vi "Engineering mode.vi"() -> ()   [LabVIEW 2017]
uses:
  Ctrls/TesterInfo.ctl
  Ctrls/control_hard.ctl
  Ctrls/HD Config.ctl
  Ctrls/AllControls.ctl
  <vilib>/Utility/miscctls.llb/LVRowAndColumnTypeDef.ctl
  Ctrls/Position Config.ctl
  Thorlabs.MotionControl.IntegratedStepperMotorsCLI.dll
  ComVIS/Files/Ini/WriteIniFiles_ByVarient.vi
  <vilib>/Utility/file.llb/Write Delimited Spreadsheet (string).vi
  HardWare/ADLINK/IO/Adlink IO/Adlink IO.lvlib
  Thorlabs.MotionControl.Controls.dll
panel:
  in  "Production Mode":bool
  out "Boolean":bool=TRUE
  in  "SerialNumber":string
  in  "Data":string
  out "Size":i32
  in  "AllControls":T1
  out "Save_status":string
  in  "Selecttion":T2(tab)
  in  "HD Config 2":T3
  in  "HD Config Save":bool
  in  "HD Config":T3
  in  "SW Config Save":bool
  in  "TesterInfo":T4={"Station Name"="", "Station Code"="", "ES NO."="", "Tester ID"="", "PassMark Revision"="", "Rig ID"="", "682_Tool_Repeat"="12", "Project Name"="", "FFTesterPath"=path "", "Enable_User"=FALSE, "Mode"=enum."682", "Fail_resume_mode"=FALSE}
  in  "Table":T5(tab)
  in  "Table_Data":string[][](table)
  in  "Title_Data":string[][](table)
  in  "Config":string[][](table)
  in  "SKU_Table":string[][](table)
  in  "Debug":T6
  in  "IO":i32(listbox)
  in  "LongTravelStageControl":refnum<k24>(container)
  in  "MoveAbsolute2":bool
  in  "MoveAbsolute1":bool
  in  "White":dbl=60.0 max=150.0
  in  "Home":bool
  in  "Black":dbl=30.0 max=150.0
  in  "Position Config Save":bool
  out "LedValue":string
  in  "Led_Read":bool
  out "Led Data":string
  out "standard output":string
  in  "SendCMD":bool
  in  "NFC_Connect":bool
  out "NFC_Connected":string
  in  "682_Tool_CMD":T7(ring)
  out "temperature":dbl
  out "humidity":dbl
  in  "ReadTemp&Hum":bool
  out "Res Data":string
  # "Unit: mm"
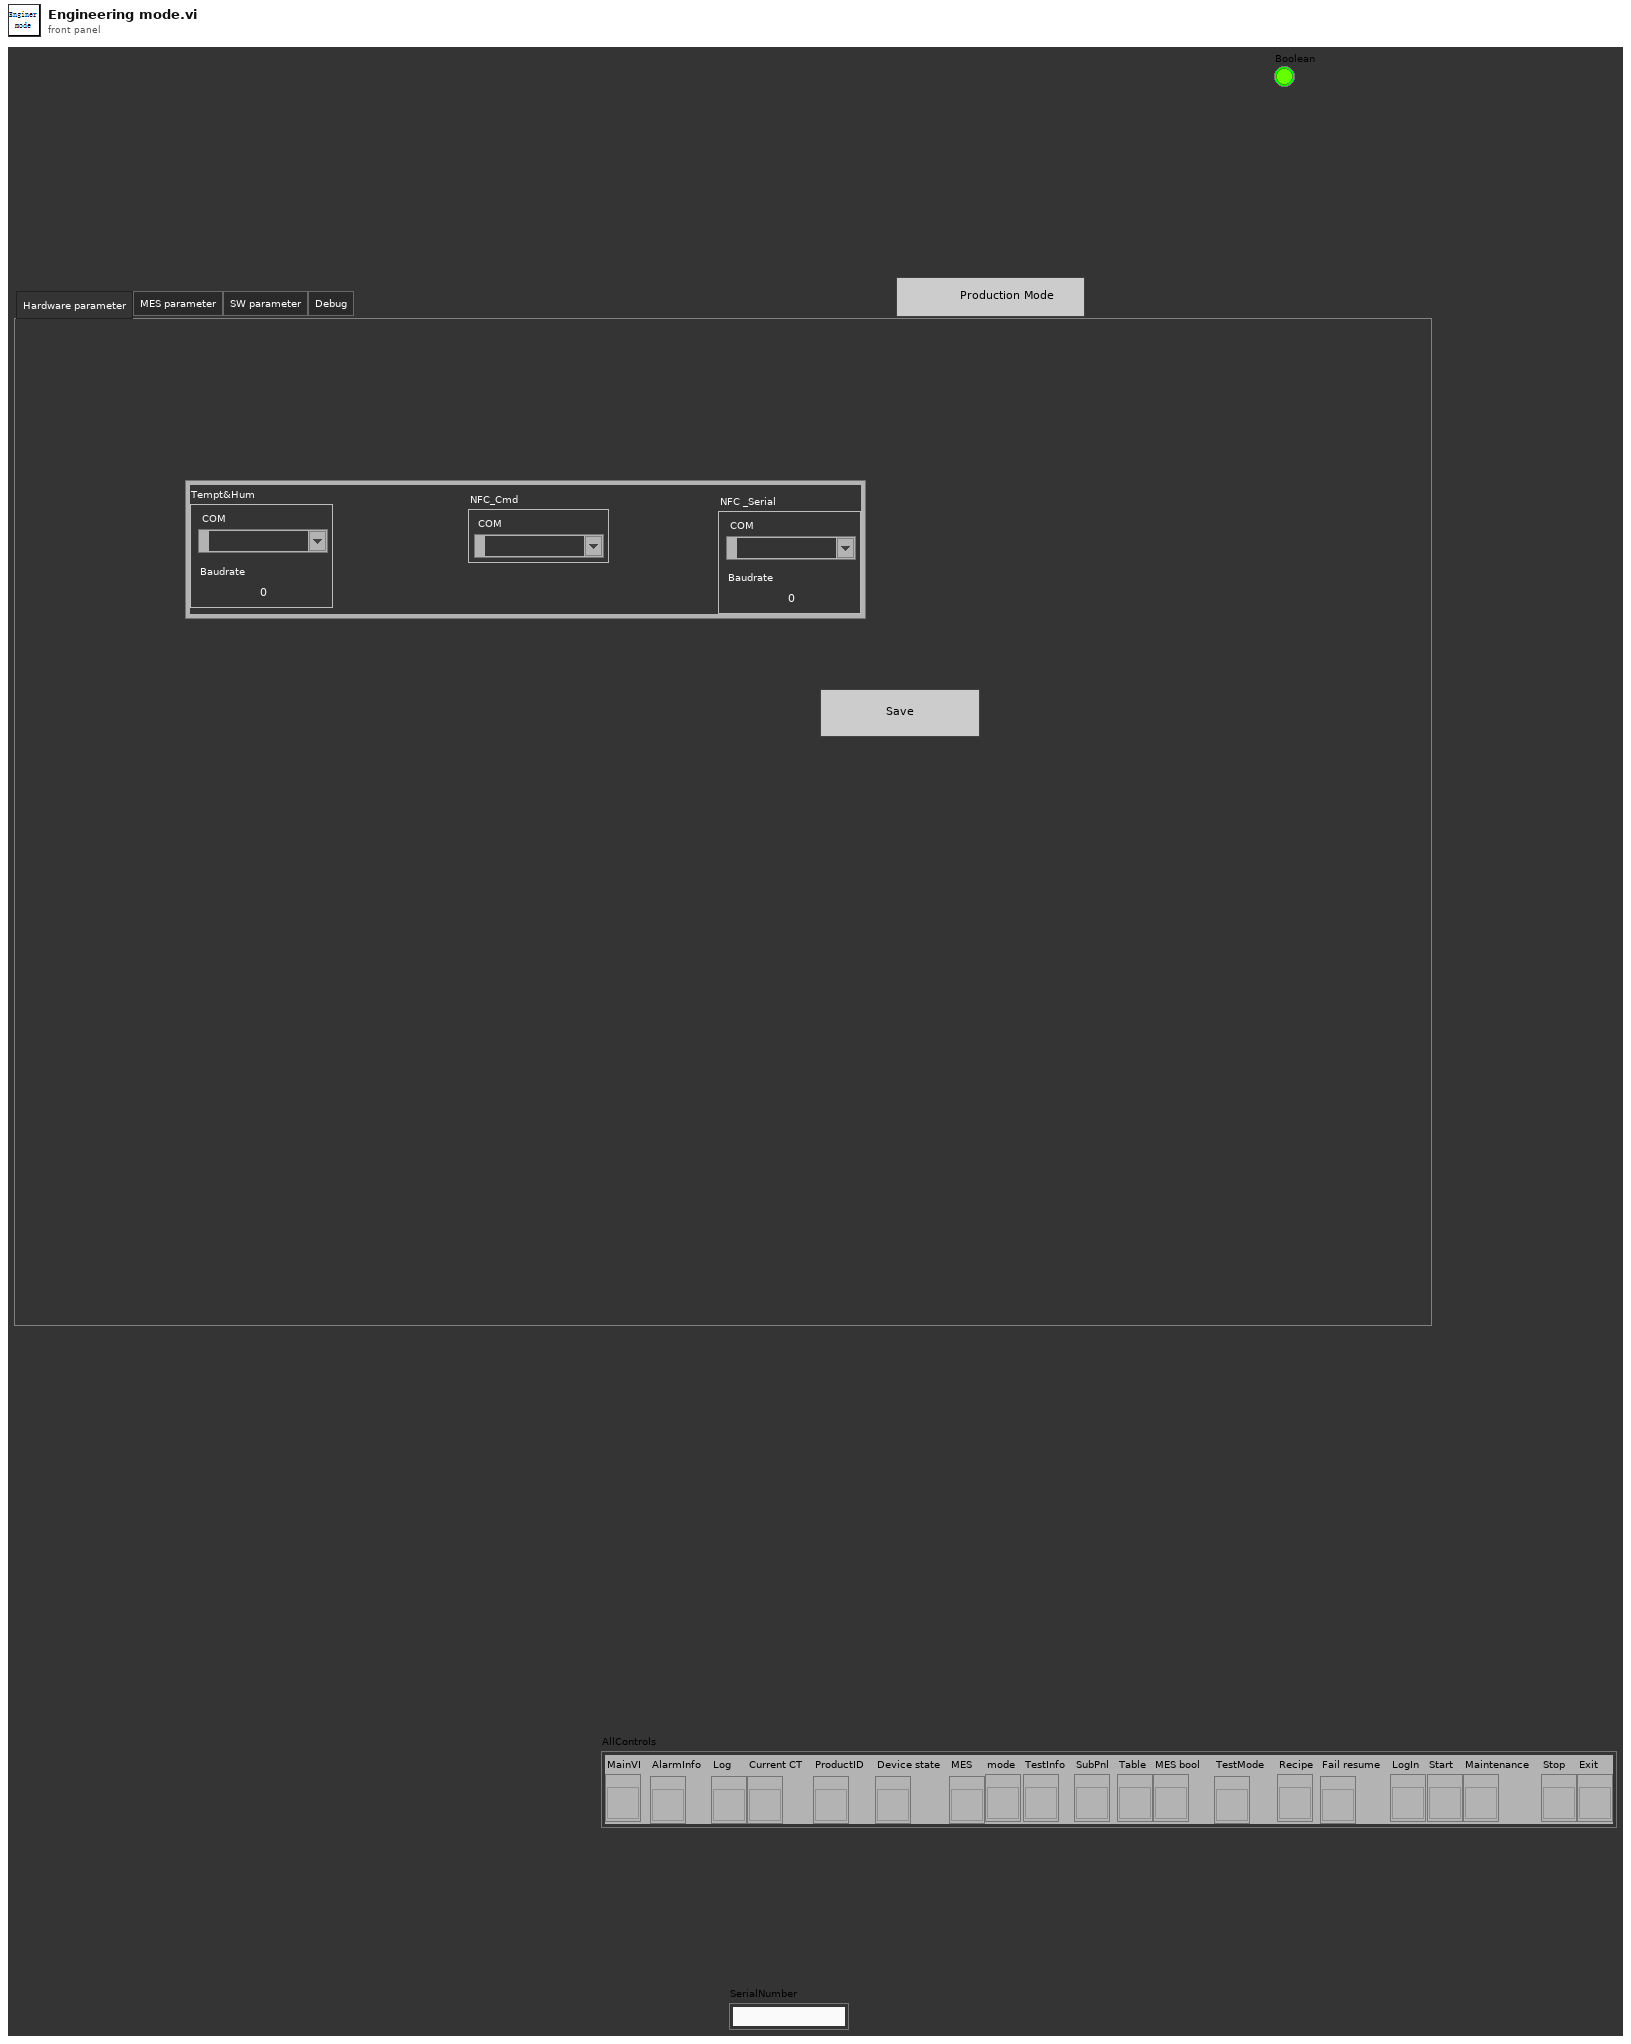
[diagram p1: front panel]
types:
  T1 = typedef "AllControls.ctl" = cluster{"MainVI":refnum<vi>, "AlarmInfo":refnum<vi>, "Log":refnum<vi>, "Current CT":refnum<vi>, "ProductID":refnum<vi>, "Device state":refnum<vi>, "MES":refnum<vi>, "mode":refnum<vi>, "TestInfo":refnum<vi>, "SubPnl":refnum<vi>, "Table":refnum<vi>, "MES bool":refnum<vi>, "TestMode":refnum<vi>, "Recipe":refnum<vi>, "Fail resume":refnum<vi>, "LogIn":refnum<vi>, "Start":refnum<vi>, "Maintenance":refnum<vi>, "Stop":refnum<vi>, "Exit":refnum<vi>}
  T2 = enum32{"Hardware parameter", "MES parameter", "SW parameter", "Debug"}
  T3 = typedef "HD Config.ctl" = cluster{" PC":cluster{"PC Address":u8[], "PC Port":i32}, "FCO":cluster{"COM":refnum<visa-resource-name>, "Baudrate":u32}, "DC Power ":cluster{"COM":refnum<visa-resource-name>, "Baudrate":u32}, "PW3336":cluster{"COM":refnum<visa-resource-name>, "Baudrate":u32}, "Lefoo":cluster{"COM":refnum<visa-resource-name>, "Baudrate":u32}, "Tempt&Hum":cluster{"COM":refnum<visa-resource-name>, "Baudrate":u32}, "DIPC":cluster{"COM":refnum<visa-resource-name>}, "Daemon":cluster{"IP Address":string, "Port":u16, "Retry":u16}, "NFC_Cmd":cluster{"COM":refnum<visa-resource-name>, "Baudrate":u32}, "Fail_resume_mode":bool, "GRR":bool, "NFC _Serial":cluster{"COM":refnum<visa-resource-name>, "Baudrate":u32}}
  T4 = typedef "TesterInfo.ctl" = cluster{"Station Name":string, "Station Code":string, "ES NO.":string, "Tester ID":string, "PassMark Revision":string, "Rig ID":string, "682_Tool_Repeat":string, "Project Name":string, "FFTesterPath":path, "Enable_User":bool, "Mode":enum16{"682"}, "Fail_resume_mode":bool}
  T5 = enum32{"Process_parameter_Setting", "Passmark_Setting", "Setting_Config", "SKU_Table"}
  T6 = typedef "control_hard.ctl" = enum32{"IO Control", "Motor_Plate control", "Led Read", "NFC ", "PW3336_Power Meter", "Lefoo_Atm Pressure", "Temp&Hum", "Set EOL_URAT"}
  T7 = enum16{"Start Test Mode", "Getting Software Version", "Start camera test mode", "Get one image", "Stop camera test mode", "Stop Test Mode", "Get image uniformity andFlash LED brightness", "Get image reflection", "Enable flash LED", "Disable flash LED", "Tune Flash LED brightness", "Start Camera calibration", "Software Reset", "Verify OBC Setting"}
  T8 = cluster{"COM":refnum<visa-resource-name>, "Baudrate":u32}
  T9 = cluster{"DI dev":i32[], "DI line":i32[], "Port":i32[], "DO dev":i32[], "DO line":i32[], "IO Data":string[][], "IO f":i16[]}
  T10 = typedef "amc_Message Queue.ctl" = refnum<queue>
  T11 = typedef "LVRowAndColumnTypeDef.ctl" = cluster{"Row":i32, "Column":i32}
  T12 = typedef "LVPoint32TypeDef.ctl" = cluster{"Horizontal":i32, "Vertical":i32}
  T13 = enum8{"Enabled", "Disabled", "Disabled and Grayed Out"}
  T14 = typedef "Position Config.ctl" = cluster{"Black":dbl, "White":dbl, "Black1":dbl, "White1":dbl}
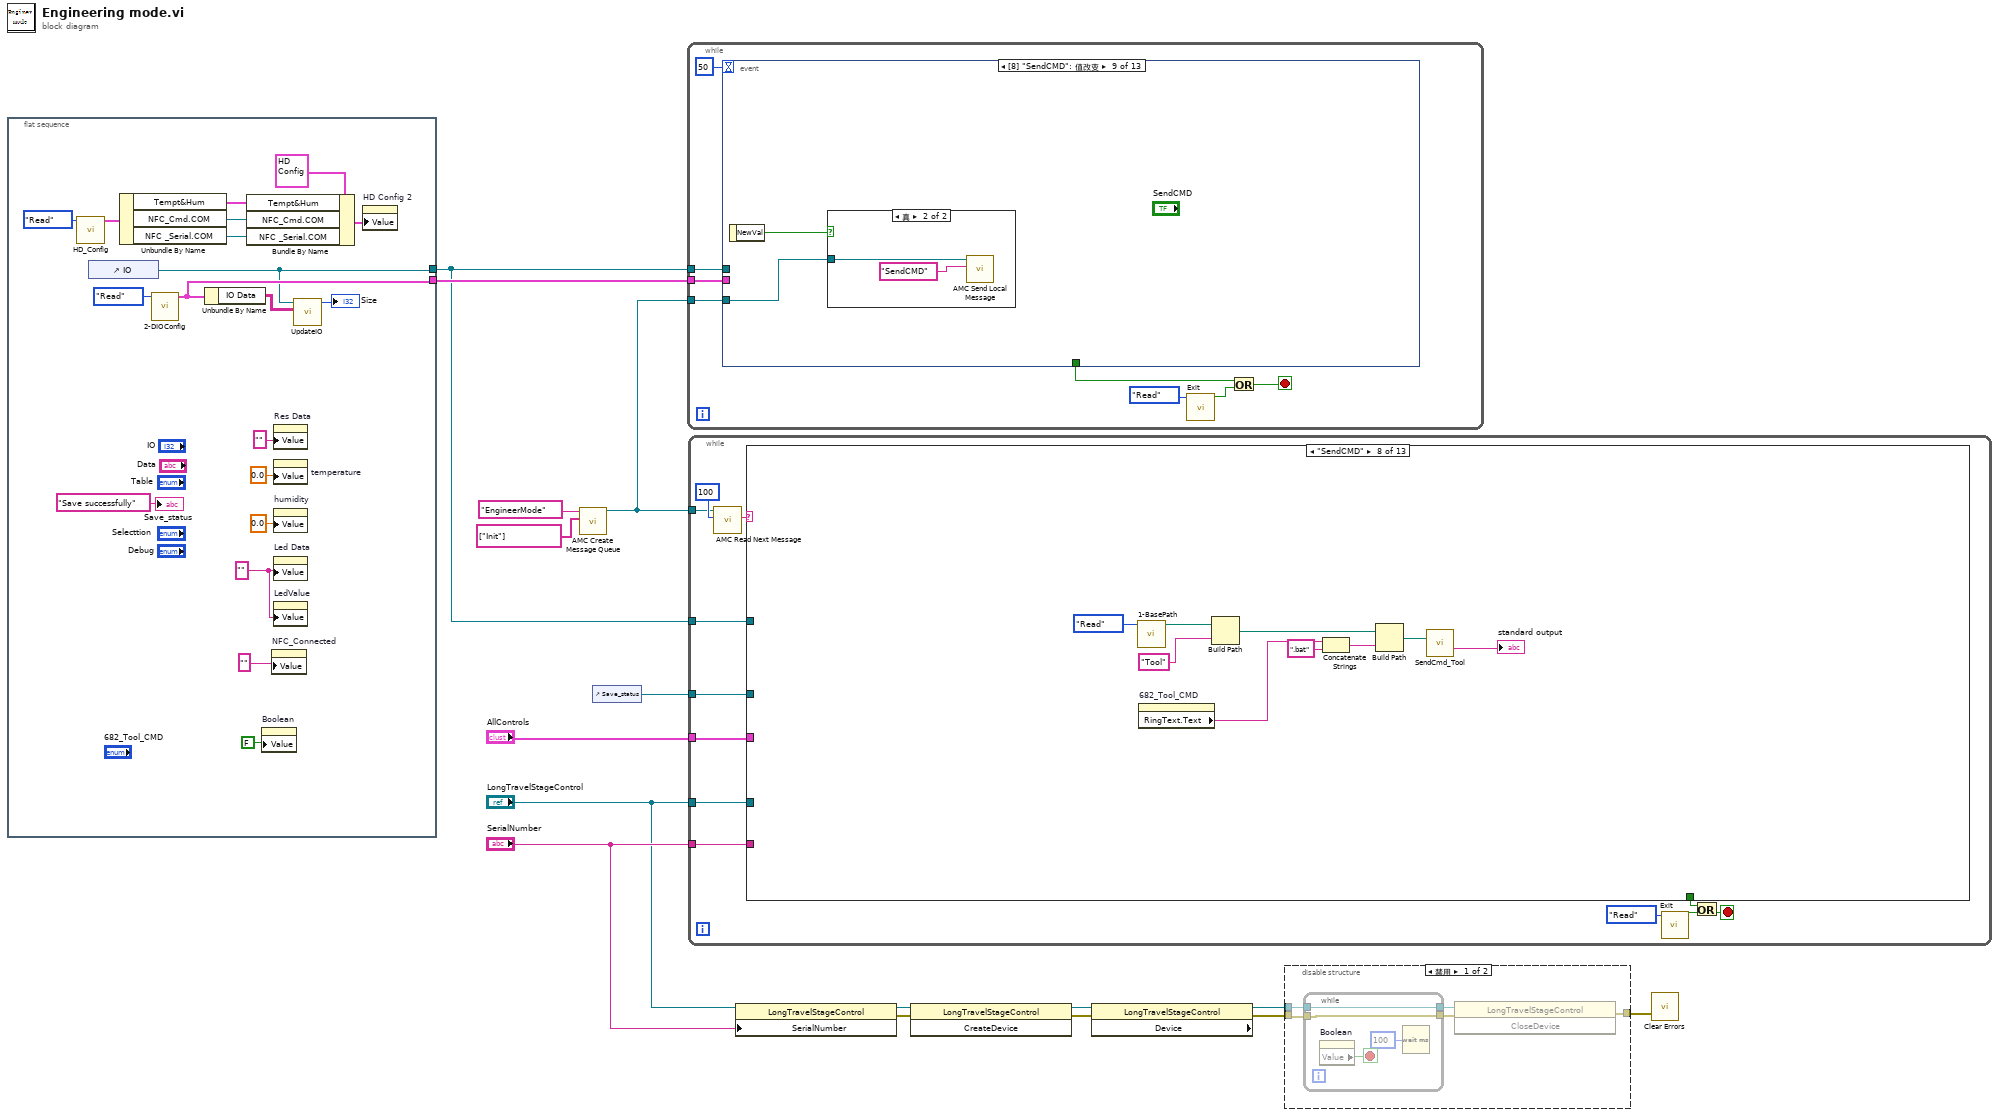
[diagram p0: block diagram]
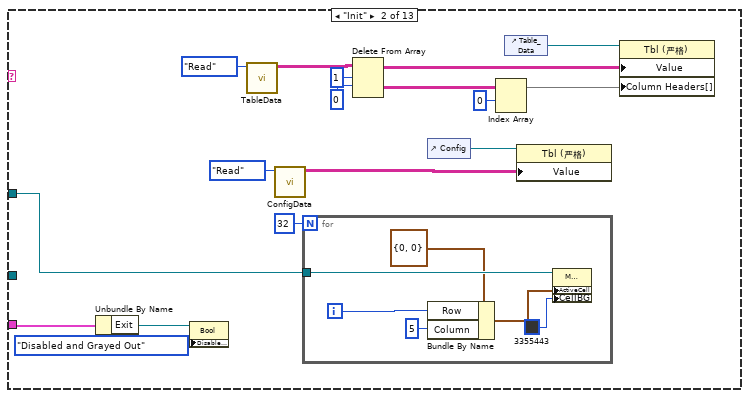
[diagram p4: hidden frame]
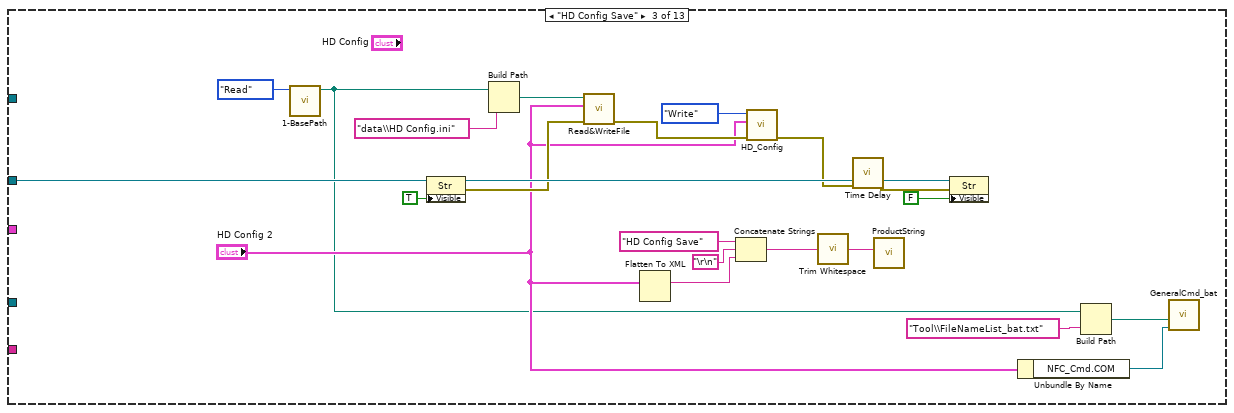
[diagram p5: hidden frame]
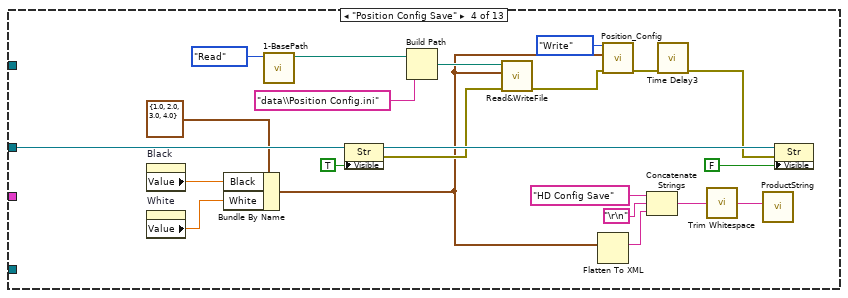
[diagram p6: hidden frame]
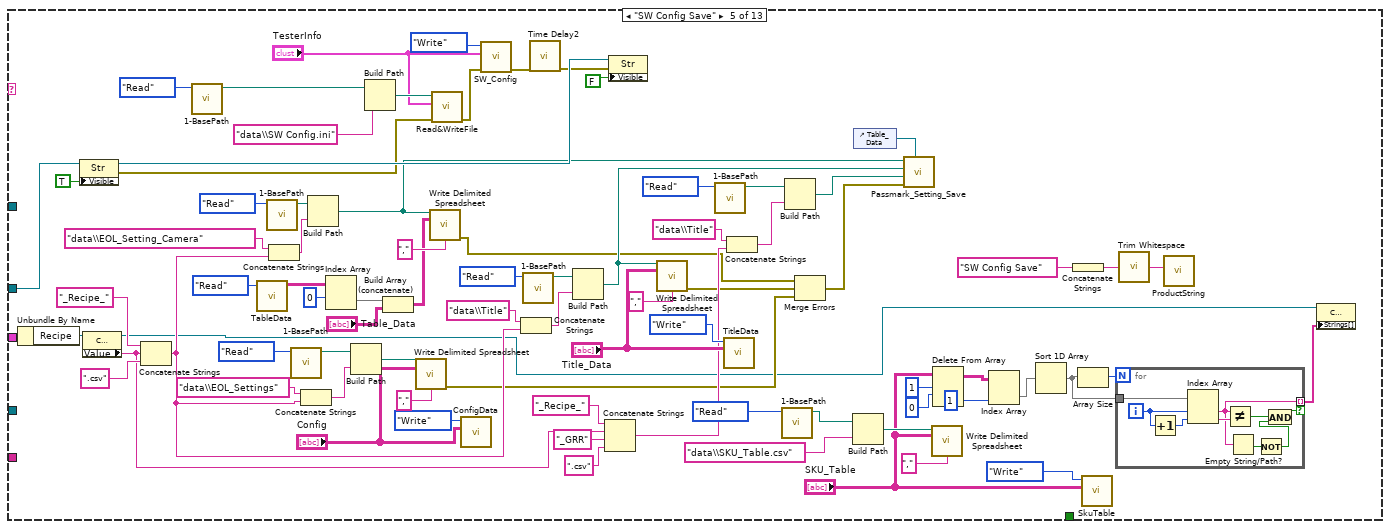
[diagram p7: hidden frame]
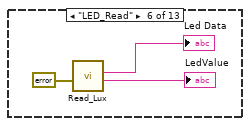
[diagram p8: hidden frame]
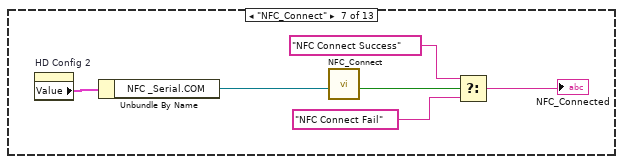
[diagram p9: hidden frame]
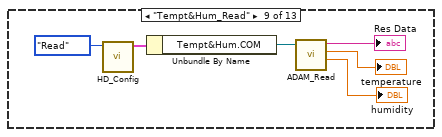
[diagram p10: hidden frame]
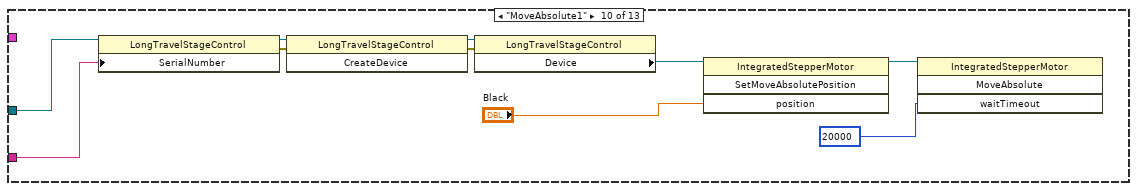
[diagram p11: hidden frame]
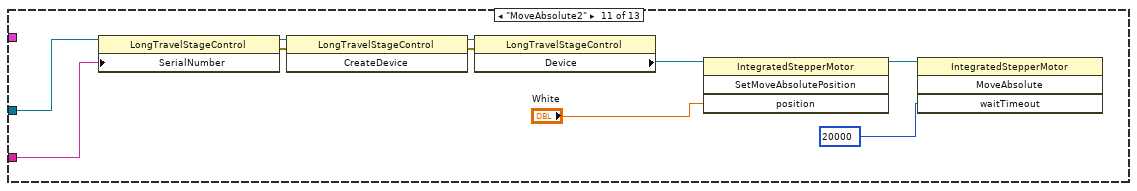
[diagram p12: hidden frame]
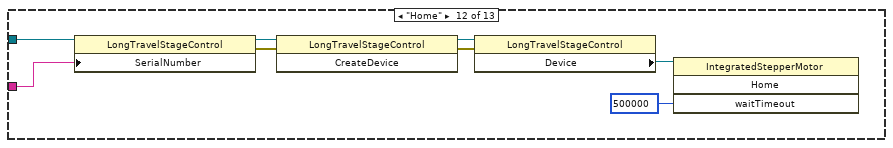
[diagram p13: hidden frame]
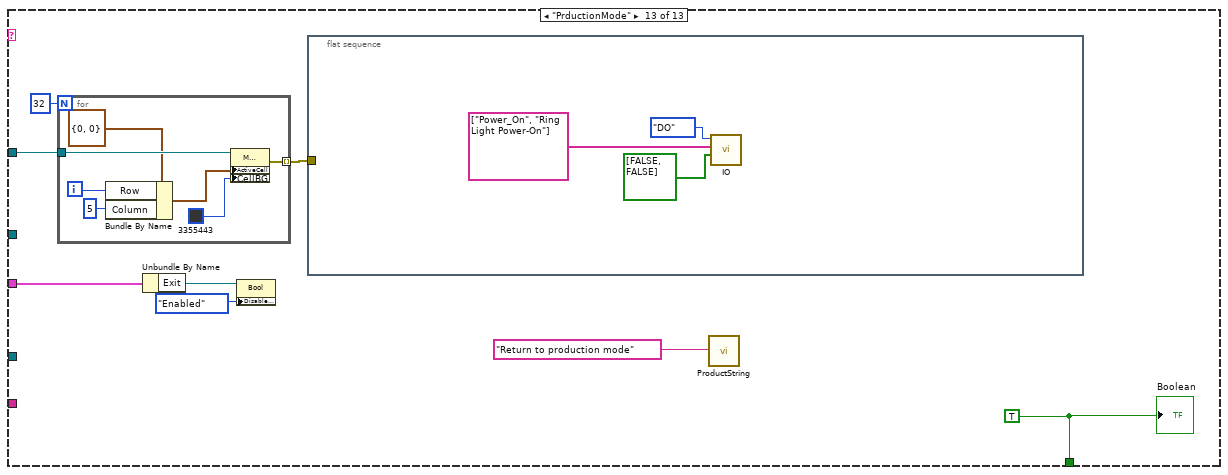
[diagram p14: hidden frame]
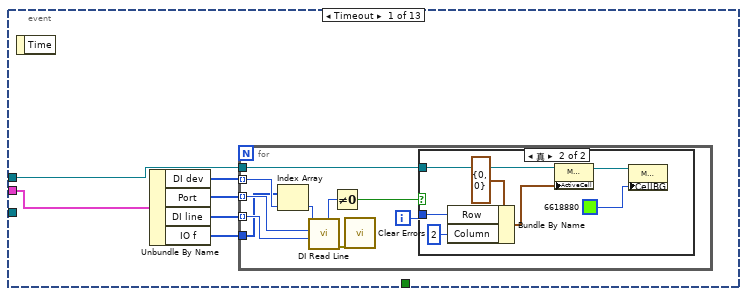
[diagram p15: hidden frame]
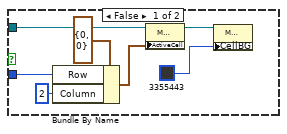
[diagram p16: hidden frame]
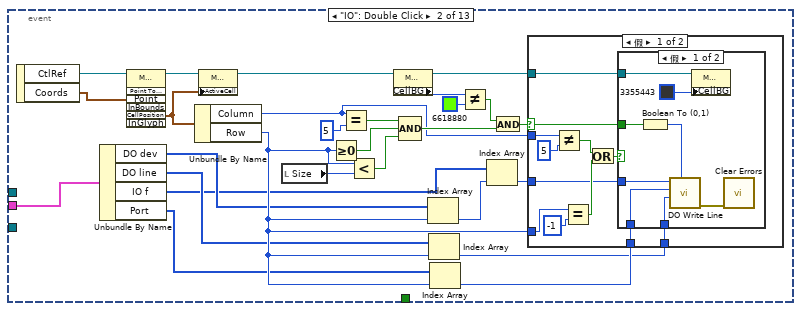
[diagram p17: hidden frame]
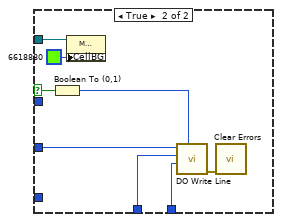
[diagram p19: hidden frame]
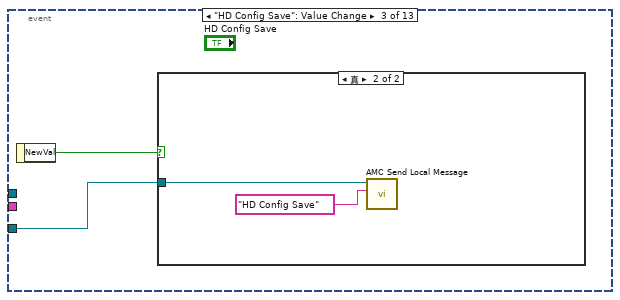
[diagram p20: hidden frame]
diagram:
  n1 = flat-sequence {
    tunnel: [w33] -> w11
    tunnel: [w31] -> w10
    frame #0 {
      w21 = "" ("Led Data")
      n2 = call "HD_Config.vi"("Step"=enum16{"Initial", "Write", "Read"}."Read") -> ("HD Config out"=w29:T3)  [unwired: 9 in, 1 out]
      n3 = control-ref of="IO"() -> (w31:refnum<vi>)
      n4 = Unbundle By Name(w29) -> ("Tempt&Hum"=w26:T8, "NFC_Cmd.COM"=w20:refnum<visa-resource-name>, "NFC _Serial.COM"=w18:refnum<visa-resource-name>)
      n5 = call "2-DIOConfig.vi"("Step"=enum16{"Initial", "Write", "Read"}."Read") -> ("DIO pra out"=w33:T9)  [unwired: 9 in, 1 out]
      n6 = Unbundle By Name(w33) -> ("IO Data"=w32:string[][])
      n7 = Bundle By Name(cluster=T3 {" PC"={"PC Address"=[], "PC Port"=0}, "FCO"={"COM"="", "Baudrate"=0}, "DC Power "={"COM"="", "Baudrate"=0}, "PW3336"={"COM"="", "Baudrate"=0}, "Lefoo"={"COM"="", "Baudrate"=0}, "Tempt&Hum"={"COM"="", "Baudrate"=0}, "DIPC"={"COM"=""}, "Daemon"={"IP Address"="", "Port"=0, "Retry"=0}, "NFC_Cmd"={"COM"="", "Baudrate"=0}, "Fail_resume_mode"=FALSE, "GRR"=FALSE, "NFC _Serial"={"COM"="", "Baudrate"=0}} ("HD Config 2"), "Tempt&Hum"=w26, "NFC_Cmd.COM"=w20, "NFC _Serial.COM"=w18) -> (w25:T3)
      n8 = property on="Boolean" class="Bool (严格)"("Value"=FALSE ("Boolean")) -> ()  [unwired: 2 in, 2 out]
      n9 = property on="NFC_Connected" class="Str"("Value"="" ("concatenated string")) -> ()  [unwired: 2 in, 2 out]
      n10 = property on="Res Data" class="Str"("Value"="" ("Res Data")) -> ()  [unwired: 2 in, 2 out]
      n11 = property on="temperature" class="DigNum (严格)"("Value"=0.0 ("temperature")) -> ()  [unwired: 2 in, 2 out]
      n12 = property on="humidity" class="DigNum (严格)"("Value"=0.0 ("humidity")) -> ()  [unwired: 2 in, 2 out]
      n13 = property on="Led Data" class="Str"("Value"=w21) -> ()  [unwired: 2 in, 2 out]
      n14 = property on="LedValue" class="Str"("Value"=w21) -> ()  [unwired: 2 in, 2 out]
      n15 = call "UpdateIO.vi"("IO Data"=w32, "MulticolumnListbox输入"=w31) -> ("大小"=→"Size":i32)  [unwired: 9 in]
      n16 = property on="HD Config 2" class="Clust (严格)"("Value"=w25) -> ()  [unwired: 2 in, 2 out]
      "Save_status" <- "Save successfully" ("Save_status")
    }
  }
  n17 = call "AMC Create Message Queue.vi"("Initial Message Names"=string[] ["Init"], "Message Queue Name"="EngineerMode" ("Message queue name (unnamed)")) -> ("Message Queue out"=w15:T10)  [unwired: 3 in, 6 out]
  n18 = control-ref of="Save_status"() -> (w14:refnum<vi>)
  n19 = while {
    tunnel: w15 -> [w40]
    tunnel: w10 -> [w38]
    tunnel: w11 -> [w37]
    stop <- w36 stop-if-true
    n20 = event shown="[8] \"SendCMD\": 值改变" {
      selector: _ -> [_ _ _ _ _ _ _ _ _ _ _ _ _]
      dyn-events: _ -> [_ _ _ _ _ _ _ _ _ _ _ _ _]
      timeout: 50 -> [_ _ _ _ _ _ _ _ _ _ _ _ _]
      tunnel: w40 -> [_ _ w130 w133 w138 w143 w150 w154 w158 w161 w165 w169 w174]
      tunnel: [_ _ _ _ _ _ _ _ _ _ _ _ w173] -> w39
      tunnel: w38 -> [w44 _ _ _ _ _ _ _ _ _ _ _ _]
      tunnel: w37 -> [w45 w76 _ _ _ _ _ _ _ _ _ _ _]
      event Timeout {
        n21 = event-data() -> ()  [unwired: 1 in, 1 out]
        n22 = Unbundle By Name(w45) -> ("DI dev"=w46:i32[], "Port"=w47:i32[], "DI line"=w48:i32[], "IO f"=w49:i16[])
        n23 = for {
          tunnel: w44 -> [w55]
          tunnel: w46 -> [w52] mode=indexing
          tunnel: w48 -> [w56] mode=indexing
          tunnel: w47 -> [w53] mode=indexing
          tunnel: w49 -> [w50]
          i -> [w54]
          n24 = Index Array(array=w50, index=w52) -> (element=w51:i16)
          n25 = call "DI Read Line.vi"("Line"=w56, "Port"=w53, "CardNumber"=w51) -> ("error out"=w59:errorcluster, "State out"=w58:u16)  [unwired: 6 in, 1 out]
          n26 = Not Equal To 0?(x=w58) -> (x != 0?=w57:bool)
          n27 = call <vilib>:"Clear Errors.vi"("error in (no error)"=w59) -> ()  [unwired: 5 in, 2 out]
          n28 = case shown="真" w57 {
            tunnel: w54 -> [w61 w70]
            tunnel: w55 -> [w60 w67]
            frame False {
              n29 = Bundle By Name(cluster=T11 {"Row"=0, "Column"=0} ("活动单元格:活动单元格"), "Row"=w61, "Column"=2) -> (w64:T11)
              n30 = property class="MCListbox (严格)"(reference=w60, "ActiveCell"=w64) -> (reference out=w66:refnum<vi>)  [unwired: 1 in, 1 out]
              n31 = property class="MCListbox (严格)"(reference=w66, "CellBG"=u32 3355443) -> ()  [unwired: 1 in, 2 out]
            }
            frame True {
              n32 = Bundle By Name(cluster=T11 {"Row"=0, "Column"=0} ("活动单元格:活动单元格"), "Row"=w70, "Column"=2) -> (w71:T11)
              n33 = property class="MCListbox (严格)"(reference=w67, "ActiveCell"=w71) -> (reference out=w73:refnum<vi>)  [unwired: 1 in, 1 out]
              n34 = property class="MCListbox (严格)"(reference=w73, "CellBG"=u32 6618880) -> ()  [unwired: 1 in, 2 out]
            }
          }
        }
      }
      event "IO": Double Click {
        n35 = event-data() -> ("CtlRef"=w75:refnum<vi>, "Coords"=w74:T12)  [unwired: 1 in]
        n36 = Unbundle By Name(w76) -> ("DO dev"=w81:i32[], "DO line"=w80:i32[], "IO f"=w79:i16[], "Port"=w98:i32[])
        n37 = invoke class="MCListbox (严格)" method="Point To Row Column"(reference=w75, "Point"=w74) -> (reference out=w94:refnum<vi>, "CellPosition"=w85:T11)  [unwired: 5 in, 5 out]
        n38 = Unbundle By Name(w85) -> ("Column"=w82:i32, "Row"=w99:i32)
        n39 = property class="MCListbox (严格)"(reference=w94, "ActiveCell"=w85) -> (reference out=w93:refnum<vi>)  [unwired: 1 in, 1 out]
        n40 = local read "Size"() -> (w84:i32)
        n41 = Greater Or Equal To 0?(x=w99) -> (x >= 0?=w90:bool)
        n42 = Equal?(x=w82, y=5) -> (x = y?=w91:bool)
        n43 = Less?(x=w99, y=w84) -> (x < y?=w83:bool)
        n44 = property class="MCListbox (严格)"(reference=w93) -> (reference out=w86:refnum<vi>, "CellBG"=w88:u32)  [unwired: 1 in, 1 out]
        n45 = Compound Arithmetic op=AND(w91, w90, w83) -> (w92:bool)
        n46 = Index Array(array=w81, index=w99) -> (element=w95:i32)
        n47 = Index Array(array=w80, index=w99) -> (element=w97:i32)
        n48 = Index Array(array=w98, index=w99) -> (element=w100:i32)
        n49 = Not Equal?(x=w88, y=u32 6618880) -> (x != y?=w89:bool)
        n50 = Index Array(array=w79, index=w95) -> (element=w96:i16)
        n51 = And(x=w89, y=w92) -> (x .and. y?=w87:bool)
        n52 = case shown="假" w87 {
          selector: w87 -> [w109 w124]
          tunnel: w86 -> [w112 w128]
          tunnel: w82 -> [w108 _]
          tunnel: w96 -> [w103 w126]
          tunnel: w97 -> [w102 w125]
          tunnel: w99 -> [w104 _]
          tunnel: w100 -> [w101 w121]
          frame False {
            n53 = Not Equal?(x=w108, y=5) -> (x != y?=w105:bool)
            n54 = Equal?(x=w104, y=-1) -> (x = y?=w110:bool)
            n55 = Or(x=w105, y=w110) -> (x .or. y?=w106:bool)
            n56 = case shown="假" w106 {
              tunnel: w112 -> [w119 _]
              tunnel: w109 -> [w114 _]
              tunnel: w103 -> [w115 _]
              tunnel: w102 -> [w116 _]
              tunnel: w101 -> [w113 _]
              frame False {
                n57 = Boolean To (0,1)(Boolean=w114) -> (0, 1=w118:i16)
                n58 = call "DO Write Line.vi"("Value"=w118, "Line"=w116, "Port"=w113, "CardNumber"=w115) -> ("error out"=w117:errorcluster)  [unwired: 6 in, 1 out]
                n59 = property class="MCListbox (严格)"(reference=w119, "CellBG"=u32 3355443) -> ()  [unwired: 1 in, 2 out]
                n60 = call <vilib>:"Clear Errors.vi"("error in (no error)"=w117) -> ()  [unwired: 5 in, 2 out]
              }
              frame True {
              }
            }
          }
          frame True {
            n61 = Boolean To (0,1)(Boolean=w124) -> (0, 1=w123:i16)
            n62 = property class="MCListbox (严格)"(reference=w128, "CellBG"=u32 6618880) -> ()  [unwired: 1 in, 2 out]
            n63 = call "DO Write Line.vi"("Value"=w123, "Line"=w125, "Port"=w121, "CardNumber"=w126) -> ("error out"=w122:errorcluster)  [unwired: 6 in, 1 out]
            n64 = call <vilib>:"Clear Errors.vi"("error in (no error)"=w122) -> ()  [unwired: 5 in, 2 out]
          }
        }
      }
      event "HD Config Save": Value Change {
        n65 = event-data() -> ("NewVal"=w129:bool)  [unwired: 1 in]
        n66 = case shown="真" w129 {
          tunnel: w130 -> [_ w132]
          frame False {
          }
          frame True {
            n67 = call "AMC Send Local Message.vi"("Message Name"="HD Config Save", "Message Queue in"=w132) -> ()  [unwired: 8 in, 2 out]
          }
        }
      }
      event "SW Config Save": Value Change {
        n68 = event-data() -> ("NewVal"=w134:bool)  [unwired: 1 in]
        n69 = case shown="真" w134 {
          tunnel: w133 -> [_ w136]
          frame False {
          }
          frame True {
            n70 = call "AMC Send Local Message.vi"("Message Name"="SW Config Save", "Message Queue in"=w136) -> ()  [unwired: 8 in, 2 out]
          }
        }
      }
      event "Position Config Save": Value Change {
        n71 = event-data() -> ("NewVal"=w137:bool)  [unwired: 1 in]
        n72 = case shown="真" w137 {
          tunnel: w138 -> [_ w140]
          frame False {
          }
          frame True {
            n73 = call "AMC Send Local Message.vi"("Message Name"="Position Config Save", "Message Queue in"=w140) -> ()  [unwired: 8 in, 2 out]
          }
        }
      }
      event "Led_Read": Value Change {
        w141 = "" ("Led Data")
        n74 = event-data() -> ("NewVal"=w142:bool)  [unwired: 1 in]
        n75 = case shown="真" w142 {
          tunnel: w143 -> [_ w144]
          frame False {
          }
          frame True {
            n76 = call "AMC Send Local Message.vi"("Message Name"="LED_Read", "Message Queue in"=w144) -> ()  [unwired: 8 in, 2 out]
          }
        }
        n77 = property on="Led Data" class="Str"("Value"=w141) -> ()  [unwired: 2 in, 2 out]
        n78 = property on="LedValue" class="Str"("Value"=w141) -> ()  [unwired: 2 in, 2 out]
      }
      event "ReadTemp&Hum": Value Change {
        n79 = event-data() -> ("NewVal"=w149:bool)  [unwired: 1 in]
        n80 = case shown="真" w149 {
          tunnel: w150 -> [_ w151]
          frame False {
          }
          frame True {
            n81 = call "AMC Send Local Message.vi"("Message Name"="Tempt&Hum_Read", "Message Queue in"=w151) -> ()  [unwired: 8 in, 2 out]
          }
        }
        n82 = property on="Res Data" class="Str"("Value"="" ("Res Data")) -> ()  [unwired: 2 in, 2 out]
        n83 = property on="temperature" class="DigNum (严格)"("Value"=0.0 ("temperature")) -> ()  [unwired: 2 in, 2 out]
        n84 = property on="humidity" class="DigNum (严格)"("Value"=0.0 ("humidity")) -> ()  [unwired: 2 in, 2 out]
      }
      event "NFC_Connect": Value Change {
        n85 = event-data() -> ("NewVal"=w153:bool)  [unwired: 1 in]
        n86 = case shown="真" w153 {
          tunnel: w154 -> [_ w155]
          frame False {
          }
          frame True {
            n87 = call "AMC Send Local Message.vi"("Message Name"="NFC_Connect", "Message Queue in"=w155) -> ()  [unwired: 8 in, 2 out]
          }
        }
      }
      event "SendCMD": Value Change {
        n88 = event-data() -> ("NewVal"=w157:bool)  [unwired: 1 in]
        n89 = case shown="真" w157 {
          tunnel: w158 -> [_ w159]
          frame False {
          }
          frame True {
            n90 = call "AMC Send Local Message.vi"("Message Name"="SendCMD", "Message Queue in"=w159) -> ()  [unwired: 8 in, 2 out]
          }
        }
      }
      event "MoveAbsolute1": Value Change {
        n91 = event-data() -> ("NewVal"=w162:bool)  [unwired: 1 in]
        n92 = case shown="真" w162 {
          tunnel: w161 -> [_ w164]
          frame False {
          }
          frame True {
            n93 = call "AMC Send Local Message.vi"("Message Name"="MoveAbsolute1", "Message Queue in"=w164) -> ()  [unwired: 8 in, 2 out]
          }
        }
      }
      event "MoveAbsolute2": Value Change {
        n94 = event-data() -> ("NewVal"=w166:bool)  [unwired: 1 in]
        n95 = case shown="真" w166 {
          tunnel: w165 -> [_ w168]
          frame False {
          }
          frame True {
            n96 = call "AMC Send Local Message.vi"("Message Name"="MoveAbsolute2", "Message Queue in"=w168) -> ()  [unwired: 8 in, 2 out]
          }
        }
      }
      event "Home": Value Change {
        n97 = event-data() -> ("NewVal"=w170:bool)  [unwired: 1 in]
        n98 = case shown="真" w170 {
          tunnel: w169 -> [_ w172]
          frame False {
          }
          frame True {
            n99 = call "AMC Send Local Message.vi"("Message Name"="Home", "Message Queue in"=w172) -> ()  [unwired: 8 in, 2 out]
          }
        }
      }
      event "Production Mode": Value Change {
        n100 = event-data() -> ("NewVal"=w175:bool)  [unwired: 1 in]
        n101 = case shown="真" w175 {
          tunnel: w174 -> [_ w177]
          tunnel: [_ TRUE ("停止")] -> w173
          frame False {
          }
          frame True {
            n102 = call "AMC Send Local Message.vi"("Message Name"="PrductionMode", "Message Queue in"=w177) -> ()  [unwired: 8 in, 2 out]
          }
        }
      }
    }
    n103 = call "Exit.vi"("Step"=enum16{"Initial", "Write", "Read"}."Read") -> ("Exit Out"=w42:bool)  [unwired: 9 in, 1 out]
    n104 = Or(x=w39, y=w42) -> (x .or. y?=w36:bool)
  }
  n105 = while {
    tunnel: w15 -> [w187]
    tunnel: w14 -> [w183]
    tunnel: "AllControls" -> [w182]
    tunnel: w10 -> [w181]
    tunnel: "LongTravelStageControl" -> [w180]
    tunnel: "SerialNumber" -> [w179]
    stop <- w185 stop-if-true
    n106 = call "AMC Read Next Message.vi"("timeout (1ms)"=100 ("Timeout"), "Message Queue in"=w187) -> ("Message Name"=w186:string)  [unwired: 2 in, 7 out]
    n107 = case shown="\"SendCMD\"" w186 {
      tunnel: [_ _ _ _ _ _ _ _ _ _ _ _ w407] -> w184
      tunnel: w183 -> [_ _ w227 w249 w335 _ _ _ _ _ _ _ _]
      tunnel: w182 -> [_ w193 _ _ w302 _ _ _ _ _ _ _ w401]
      tunnel: w181 -> [_ w194 _ _ _ _ _ _ _ _ _ _ w406]
      tunnel: w180 -> [_ _ _ _ _ _ _ _ _ w373 w384 w395 _]
      tunnel: w179 -> [_ _ _ _ _ _ _ _ _ w372 w383 w394 _]
      frame "假", Default {
      }
      frame "Init" {
        n108 = Unbundle By Name(w193) -> ("Exit"=w192:refnum<vi>)
        n109 = property class="Bool"(reference=w192, "DisabledEnum"=T13."Disabled and Grayed Out" ("Disabled")) -> ()  [unwired: 1 in, 2 out]
        n110 = call "TableData.vi"("Step"=enum16{"Initial", "Write", "Read"}."Read") -> ("Tabledata Out"=w203:string[][])  [unwired: 9 in, 1 out]
        n111 = call "ConfigData.vi"("Step"=enum16{"Initial", "Write", "Read"}."Read") -> ("Tabledata Out"=w196:string[][])  [unwired: 9 in, 1 out]
        n112 = for {
          N: 32 -> [_]
          tunnel: w194 -> [w213]
          i -> [w209]
          n113 = Bundle By Name(cluster=T11 {"Row"=0, "Column"=0} ("Active Cell:Active Cell"), "Row"=w209, "Column"=5) -> (w210:T11)
          n114 = property class="MCListbox (严格)"(reference=w213, "ActiveCell"=w210, "CellBG"=u32 3355443) -> ()  [unwired: 1 in, 2 out]
        }
        n115 = Delete From Array(array=w203, length=1 ("长度"), index (row)=0 ("索引 (行)")) -> (deleted portion=w201:string[][], array with subset deleted=w202:string[][])  [unwired: 1 in]
        n116 = control-ref of="Config"() -> (w197:refnum<vi>)
        n117 = Index Array(array=w201, index (row)=0 ("索引 (行)")) -> (element=w200:string[])  [unwired: 1 in]
        n118 = control-ref of="Table_Data"() -> (w207:refnum<vi>)
        n119 = property on="属性节点" class="Tbl (严格)"(reference=w197, "Value"=w196) -> ()  [unwired: 1 in, 2 out]
        n120 = property on="属性节点" class="Tbl (严格)"(reference=w207, "Value"=w202, "Column Headers[]"=w200) -> ()  [unwired: 1 in, 2 out]
      }
      frame "HD Config Save" {
        n121 = call "1-BasePath.vi"("Step"=enum16{"Initial", "Write", "Read"}."Read") -> ("Path Out"=w214:path)  [unwired: 9 in, 1 out]
        n122 = property class="Str"(reference=w227, "Visible"=TRUE ("可见")) -> (reference out=w230:refnum<vi>, error out=w229:errorcluster)  [unwired: 1 in]
        n123 = Build Path(base path=w214, name or relative path="data\\HD Config.ini") -> (appended path=w233:path)
        n124 = call-poly "Read&WriteFile.vi"("error in (no error)"=w229, "Variant"="HD Config 2", "path"=w233) -> ("error out"=w220:errorcluster)  [unwired: 8 in]
        n125 = Flatten To XML(anything="HD Config 2") -> (xml string=w225:string)
        n126 = Concatenate Strings("HD Config Save" ("String"), "\r\n", w225) -> (w226:string)
        n127 = call "HD_Config.vi"("error in (no error)"=w220, "HD Config in"="HD Config 2", "Step"=enum16{"Initial", "Write", "Read"}."Write") -> ("error out"=w219:errorcluster)  [unwired: 7 in, 1 out]
        n128 = call <vilib>:"Trim Whitespace.vi"("string"=w226) -> ("trimmed string"=w223:string)  [unwired: 1 in]
        n129 = call "Time Delay"("error in (no error)"=w219) -> ("error out"=w221:errorcluster)  [unwired: 10 in]
        n130 = call "ProductString.vi"("String"=w223) -> ()  [unwired: 10 in, 1 out]
        n131 = property class="Str"(reference=w230, error in=w221, "Visible"=FALSE ("可见")) -> ()  [unwired: 2 out]
        n132 = Unbundle By Name("HD Config 2") -> ("NFC_Cmd.COM"=w215:refnum<visa-resource-name>)
        n133 = Build Path(base path=w214, name or relative path="Tool\\FileNameList_bat.txt") -> (appended path=w217:path)
        n134 = call "GeneralCmd_bat.vi"("COM"=w215, "fileList_bat"=w217) -> ()  [unwired: 9 in, 1 out]
      }
      frame "Position Config Save" {
        n135 = property on="Black" class="DigNum (严格)"() -> ("Value"=w238:dbl)  [unwired: 2 in, 2 out]
        n136 = property on="White" class="DigNum (严格)"() -> ("Value"=w237:dbl)  [unwired: 2 in, 2 out]
        n137 = Bundle By Name(cluster=T14 {"Black"=1.0, "White"=2.0, "Black1"=3.0, "White1"=4.0} ("Position Config"), "Black"=w238, "White"=w237) -> (w236:T14)
        n138 = call "1-BasePath.vi"("Step"=enum16{"Initial", "Write", "Read"}."Read") -> ("Path Out"=w240:path)  [unwired: 9 in, 1 out]
        n139 = property class="Str"(reference=w249, "Visible"=TRUE ("可见")) -> (reference out=w252:refnum<vi>, error out=w251:errorcluster)  [unwired: 1 in]
        n140 = Build Path(base path=w240, name or relative path="data\\Position Config.ini") -> (appended path=w255:path)
        n141 = call-poly "Read&WriteFile.vi"("error in (no error)"=w251, "Variant"=w236, "path"=w255) -> ("error out"=w243:errorcluster)  [unwired: 8 in]
        n142 = Flatten To XML(anything=w236) -> (xml string=w247:string)
        n143 = call "Position_Config.vi"("error in (no error)"=w243, "Position Config"=w236, "Step"=enum16{"Initial", "Write", "Read"}."Write") -> ("error out"=w242:errorcluster)  [unwired: 7 in, 1 out]
        n144 = Concatenate Strings("HD Config Save" ("String"), "\r\n", w247) -> (w248:string)
        n145 = call "Time Delay3"("error in (no error)"=w242) -> ("error out"=w241:errorcluster)  [unwired: 10 in]
        n146 = call <vilib>:"Trim Whitespace.vi"("string"=w248) -> ("trimmed string"=w245:string)  [unwired: 1 in]
        n147 = call "ProductString.vi"("String"=w245) -> ()  [unwired: 10 in, 1 out]
        n148 = property class="Str"(reference=w252, error in=w241, "Visible"=FALSE ("可见")) -> ()  [unwired: 2 out]
      }
      frame "SW Config Save" {
        n149 = Unbundle By Name(w302) -> ("Recipe"=w264:refnum<vi>)
        n150 = property class="Str"(reference=w335, "Visible"=TRUE ("可见")) -> (reference out=w337:refnum<vi>, error out=w327:errorcluster)  [unwired: 1 in]
        n151 = property class="CmbBox"(reference=w264) -> (reference out=w263:refnum<vi>, "Value"=w284:string)  [unwired: 1 in, 1 out]
        n152 = Concatenate Strings("_Recipe_" ("字符串"), w284, ".csv" ("字符串")) -> (w293:string)
        n153 = call "1-BasePath.vi"("Step"=enum16{"Initial", "Write", "Read"}."Read") -> ("Path Out"=w258:path)  [unwired: 9 in, 1 out]
        n154 = call "TableData.vi"("Step"=enum16{"Initial", "Write", "Read"}."Read") -> ("Tabledata Out"=w317:string[][])  [unwired: 9 in, 1 out]
        n155 = call "1-BasePath.vi"("Step"=enum16{"Initial", "Write", "Read"}."Read") -> ("Path Out"=w323:path)  [unwired: 9 in, 1 out]
        n156 = Concatenate Strings("data\\EOL_Setting_Camera" ("name or relative path"), w293) -> (w298:string)
        n157 = call "1-BasePath.vi"("Step"=enum16{"Initial", "Write", "Read"}."Read") -> ("Path Out"=w311:path)  [unwired: 9 in, 1 out]
        n158 = Concatenate Strings("data\\EOL_Settings" ("name or relative path"), w293) -> (w296:string)
        n159 = Build Path(base path=w323, name or relative path=w298) -> (appended path=w292:path)
        n160 = Index Array ("索引数组")(array=w317, index (row)=0 ("索引 (行)")) -> (element=w316:string[])  [unwired: 1 in]
        n161 = Build Path(base path=w311, name or relative path=w296) -> (appended path=w313:path)
        n162 = Build Path(base path=w258, name or relative path="data\\SW Config.ini") -> (appended path=w329:path)
        n163 = Build Array (concatenate)(w316, "Table_Data") -> (w320:string[][])
        n164 = call-poly <vilib>:"Write Delimited Spreadsheet.vi"("file path (dialog if empty)"=w313, "2D data"="Config", "delimiter (\\t)"="," ("delimiter (\\t)")) -> ("error out"=w277:errorcluster)  [unwired: 11 in, 1 out]
        n165 = call-poly <vilib>:"Write Delimited Spreadsheet.vi"("file path (dialog if empty)"=w292, "2D data"=w320, "delimiter (\\t)"="," ("delimiter (\\t)")) -> ("error out"=w276:errorcluster)  [unwired: 11 in, 1 out]
        n166 = call-poly "Read&WriteFile.vi"("error in (no error)"=w327, "Variant"="TesterInfo", "path"=w329) -> ("error out"=w326:errorcluster)  [unwired: 8 in]
        n167 = call "ConfigData.vi"("Tabledata in"="Config", "Step"=enum16{"Initial", "Write", "Read"}."Write") -> ()  [unwired: 8 in, 2 out]
        n168 = call "SW_Config.vi"("error in (no error)"=w326, "SW Config In"="TesterInfo", "Step"=enum16{"Initial", "Write", "Read"}."Write") -> ("error out"=w325:errorcluster)  [unwired: 7 in, 1 out]
        n169 = Concatenate Strings("data\\Title" ("name or relative path"), w293) -> (w294:string)
        n170 = call "1-BasePath.vi"("Step"=enum16{"Initial", "Write", "Read"}."Read") -> ("Path Out"=w305:path)  [unwired: 9 in, 1 out]
        n171 = call "Time Delay2"("error in (no error)"=w325) -> ("error out"=w309:errorcluster)  [unwired: 10 in]
        n172 = Build Path(base path=w305, name or relative path=w294) -> (appended path=w291:path)
        n173 = Concatenate Strings("_Recipe_" ("字符串"), w284, "_GRR" ("字符串"), ".csv" ("字符串")) -> (w281:string)
        n174 = property class="Str"(reference=w337, error in=w309, "Visible"=FALSE ("可见")) -> ()  [unwired: 2 out]
        n175 = call-poly <vilib>:"Write Delimited Spreadsheet.vi"("file path (dialog if empty)"=w291, "2D data"="Title_Data", "delimiter (\\t)"="," ("delimiter (\\t)")) -> ("error out"=w280:errorcluster)  [unwired: 11 in, 1 out]
        n176 = call "1-BasePath.vi"("Step"=enum16{"Initial", "Write", "Read"}."Read") -> ("Path Out"=w288:path)  [unwired: 9 in, 1 out]
        n177 = call "TitleData.vi"("Tabledata in"="Title_Data", "Step"=enum16{"Initial", "Write", "Read"}."Write") -> ()  [unwired: 8 in, 2 out]
        n178 = Concatenate Strings("data\\Title" ("name or relative path"), w281) -> (w290:string)
        n179 = call "1-BasePath.vi"("Step"=enum16{"Initial", "Write", "Read"}."Read") -> ("Path Out"=w270:path)  [unwired: 9 in, 1 out]
        n180 = Build Path(base path=w288, name or relative path=w290) -> (appended path=w286:path)
        n181 = Merge Errors(w276, w280, w277) -> (w278:errorcluster)
        n182 = Build Path(base path=w270, name or relative path="data\\SKU_Table.csv") -> (appended path=w275:path)
        n183 = control-ref of="Table_Data"() -> (w279:refnum<vi>)
        n184 = call "Passmark_Setting_Save.vi"("Table_Data 2"=w279, "error in (no error)"=w278, "GRR_Title_Setting_path"=w286, "Title_Setting_path"=w291, "Flow_Setting_path"=w292) -> ()  [unwired: 6 in, 1 out]
        n185 = call-poly <vilib>:"Write Delimited Spreadsheet.vi"("file path (dialog if empty)"=w275, "2D data"="SKU_Table", "delimiter (\\t)"="," ("delimiter (\\t)")) -> ()  [unwired: 11 in, 2 out]
        n186 = Delete From Array(array="SKU_Table", length=1 ("长度"), index (row)=0 ("索引 (行)")) -> (array with subset deleted=w269:string[][])  [unwired: 1 in, 1 out]
        n187 = Index Array(array=w269, index (col)=1 ("禁用的索引 (列)")) -> (element=w262:string[])  [unwired: 1 in]
        n188 = Sort 1D Array(array=w262) -> (sorted array=w260:string[])
        n189 = Concatenate Strings("SW Config Save" ("String")) -> (w334:string)
        n190 = Array Size(array=w260) -> (size(s)=w261:i32)
        n191 = call "SkuTable.vi"("Tabledata in"="SKU_Table", "Step"=enum16{"Initial", "Write", "Read"}."Write") -> ()  [unwired: 8 in, 2 out]
        n192 = for {
          N: w261 -> [_]
          tunnel: w260 -> [w347]
          tunnel: [w342] -> w259 mode=indexing if=w340
          i -> [w345]
          n193 = Increment(x=w345) -> (x+1=w344:i32)
          n194 = Index Array(array=w347, index #1=w345, index #2=w344) -> (element #1=w342:string, element #2=w343:string)
          n195 = Not Equal?(x=w342, y=w343) -> (x != y?=w346:bool)
          n196 = Empty String/Path?(string/path=w342) -> (empty?=w341:bool)
          n197 = Not(x=w341) -> (.not. x?=w339:bool)
          n198 = And(x=w346, y=w339) -> (x .and. y?=w340:bool)
        }
        n199 = call <vilib>:"Trim Whitespace.vi"("string"=w334) -> ("trimmed string"=w333:string)  [unwired: 1 in]
        n200 = call "ProductString.vi"("String"=w333) -> ()  [unwired: 10 in, 1 out]
        n201 = property class="CmbBox"(reference=w263, "Strings[]"=w259) -> ()  [unwired: 1 in, 2 out]
      }
      frame "LED_Read" {
        n202 = call "Read_Lux.vi"("error in (no error)"=errorcluster {"status"=FALSE, "code"=0, "source"=""} ("错误输入（无错误）")) -> ("Lux_Value"=→"LedValue":string, "ReadData"=→"Led Data":string)  [unwired: 8 in, 1 out]
      }
      frame "NFC_Connect" {
        n203 = property on="HD Config 2" class="Clust (严格)"() -> ("Value"=w356:T3)  [unwired: 2 in, 2 out]
        n204 = Unbundle By Name(w356) -> ("NFC _Serial.COM"=w355:refnum<visa-resource-name>)
        n205 = call "NFC_Connect.vi"("VISA resource name"=w355) -> ("NFC"=w354:bool)  [unwired: 9 in, 1 out]
        n206 = Select(t="NFC Connect Success", s=w354, f="NFC Connect Fail") -> (s? t:f=→"NFC_Connected":string)
      }
      frame "SendCMD" {
        n207 = call "1-BasePath.vi"("Step"=enum16{"Initial", "Write", "Read"}."Read") -> ("Path Out"=w360:path)  [unwired: 9 in, 1 out]
        n208 = property on="682_Tool_CMD" class="Enum (严格)"() -> ("RingText.Text"=w363:string)  [unwired: 2 in, 2 out]
        n209 = Build Path(base path=w360, name or relative path="Tool") -> (appended path=w364:path)
        n210 = Concatenate Strings(w363, ".bat" ("字符串")) -> (w362:string)
        n211 = Build Path(base path=w364, name or relative path=w362) -> (appended path=w361:path)
        n212 = call "SendCmd_Tool.vi"("path_bat"=w361) -> ("standard output"=→"standard output":string)  [unwired: 7 in, 7 out]
      }
      frame "Tempt&Hum_Read" {
        n213 = call "HD_Config.vi"("Step"=enum16{"Initial", "Write", "Read"}."Read") -> ("HD Config out"=w371:T3)  [unwired: 9 in, 1 out]
        n214 = Unbundle By Name(w371) -> ("Tempt&Hum.COM"=w369:refnum<visa-resource-name>)
        n215 = call "ADAM_Read.vi"("VISA resource name"=w369) -> ("humidity"=→"humidity":dbl, "temperature"=→"temperature":dbl, "Data"=→"Res Data":string)  [unwired: 7 in, 1 out]
      }
      frame "MoveAbsolute1" {
        n216 = property class="LongTravelStageControl"(reference=w373, "SerialNumber"=w372) -> (reference out=w378:refnum<k24>, error out=w380:errorcluster)  [unwired: 1 in]
        n217 = invoke class="LongTravelStageControl" method="CreateDevice"(reference=w378, error in=w380) -> (reference out=w379:refnum<k24>, error out=w381:errorcluster)  [unwired: 1 in, 1 out]
        n218 = property class="LongTravelStageControl"(reference=w379, error in=w381) -> ("Device"=w377:refnum<k24>)  [unwired: 2 out]
        n219 = invoke class="IntegratedStepperMotor" method="SetMoveAbsolutePosition"(reference=w377, "position"="Black") -> (reference out=w374:refnum<k24>)  [unwired: 2 in, 3 out]
        n220 = invoke class="IntegratedStepperMotor" method="MoveAbsolute"(reference=w374, "waitTimeout"=20000) -> ()  [unwired: 2 in, 4 out]
      }
      frame "MoveAbsolute2" {
        n221 = property class="LongTravelStageControl"(reference=w384, "SerialNumber"=w383) -> (reference out=w388:refnum<k24>, error out=w390:errorcluster)  [unwired: 1 in]
        n222 = invoke class="LongTravelStageControl" method="CreateDevice"(reference=w388, error in=w390) -> (reference out=w389:refnum<k24>, error out=w391:errorcluster)  [unwired: 1 in, 1 out]
        n223 = property class="LongTravelStageControl"(reference=w389, error in=w391) -> ("Device"=w387:refnum<k24>)  [unwired: 2 out]
        n224 = invoke class="IntegratedStepperMotor" method="SetMoveAbsolutePosition"(reference=w387, "position"="White") -> (reference out=w385:refnum<k24>)  [unwired: 2 in, 3 out]
        n225 = invoke class="IntegratedStepperMotor" method="MoveAbsolute"(reference=w385, "waitTimeout"=20000) -> ()  [unwired: 2 in, 4 out]
      }
      frame "Home" {
        n226 = property class="LongTravelStageControl"(reference=w395, "SerialNumber"=w394) -> (reference out=w397:refnum<k24>, error out=w392:errorcluster)  [unwired: 1 in]
        n227 = invoke class="LongTravelStageControl" method="CreateDevice"(reference=w397, error in=w392) -> (reference out=w398:refnum<k24>, error out=w399:errorcluster)  [unwired: 1 in, 1 out]
        n228 = property class="LongTravelStageControl"(reference=w398, error in=w399) -> ("Device"=w396:refnum<k24>)  [unwired: 2 out]
        n229 = invoke class="IntegratedStepperMotor" method="Home"(reference=w396, "waitTimeout"=500000) -> ()  [unwired: 2 in, 4 out]
      }
      frame "PrductionMode" {
        w407 = TRUE
        n230 = for {
          N: 32 -> [_]
          tunnel: w406 -> [w414]
          tunnel: [w408] -> w400 mode=indexing
          i -> [w410]
          n231 = Bundle By Name(cluster=T11 {"Row"=0, "Column"=0} ("Active Cell:Active Cell"), "Row"=w410, "Column"=5) -> (w411:T11)
          n232 = property class="MCListbox (严格)"(reference=w414, "ActiveCell"=w411, "CellBG"=u32 3355443) -> (error out=w408:errorcluster)  [unwired: 1 in, 1 out]
        }
        n233 = Unbundle By Name(w401) -> ("Exit"=w403:refnum<vi>)
        n234 = property class="Bool"(reference=w403, "DisabledEnum"=T13."Enabled" ("Disabled")) -> ()  [unwired: 1 in, 2 out]
        n235 = flat-sequence {
          tunnel: w400 -> [_]
          frame #0 {
            n236 = call "IO.vi"("DO DATA"=bool[] [FALSE, FALSE] ("Writel_IO"), "IO Name"=string[] ["Power_On", "Ring Light Power-On"], "IO?"=enum16{"DI", "DO"}."DO") -> ()  [unwired: 7 in, 2 out]
          }
        }
        n237 = call "ProductString.vi"("String"="Return to production mode") -> ()  [unwired: 10 in, 1 out]
        "Boolean" <- w407
      }
    }
    n238 = call "Exit.vi"("Step"=enum16{"Initial", "Write", "Read"}."Read") -> ("Exit Out"=w190:bool)  [unwired: 9 in, 1 out]
    n239 = Or(x=w184, y=w190) -> (x .or. y?=w185:bool)
  }
  n240 = property class="LongTravelStageControl"(reference="LongTravelStageControl", "SerialNumber"="SerialNumber") -> (reference out=w7:refnum<k24>, error out=w5:errorcluster)  [unwired: 1 in]
  n241 = invoke class="LongTravelStageControl" method="CreateDevice"(reference=w7, error in=w5) -> (reference out=w6:refnum<k24>, error out=w4:errorcluster)  [unwired: 1 in, 1 out]
  n242 = property class="LongTravelStageControl" props=["Device"](reference=w6, error in=w4) -> (reference out=w3:refnum<k24>, error out=w2:errorcluster)  [unwired: 1 out]
  n243 = disable-structure shown="禁用" {
    disable-tunnel: w3 -> [w422 _]
    disable-tunnel: w2 -> [w420 w427]
    disable-tunnel: [w418 w427] -> w1
    frame Disabled {
      n244 = while {
        tunnel: w422 -> [w426]
        tunnel: [w426] -> w421
        tunnel: [w425] -> w419
        tunnel: w420 -> [w425]
        stop <- w423 stop-if-true
        n245 = property on="Boolean" class="Bool (严格)"() -> ("Value"=w423:bool)  [unwired: 2 in, 2 out]
        n246 = Wait (ms)(milliseconds to wait=u32 100) -> ()  [unwired: 1 out]
      }
      n247 = invoke class="LongTravelStageControl" method="CloseDevice"(reference=w421, error in=w419) -> (error out=w418:errorcluster)  [unwired: 1 in, 2 out]
    }
    frame Enabled {
    }
  }
  n248 = call <vilib>:"Clear Errors.vi"("error in (no error)"=w1) -> ()  [unwired: 5 in, 2 out]
